vi "ILCTest.vi"() -> ()   [LabVIEW 2016]
uses:
  Common_RT_HPILC/DataTypes/HPTelemetry.ctl
  Stats.ctl
  Common_RT_Modbus/DataTypes/RxFrame.ctl
  Common_RT_HealthAndStatus/RTHealthAndStatus/RTHealthAndStatus.lvclass
  MyHealthAndStatusReadFIFO/MyHealthAndStatusReadFIFO.lvclass
  D:/Code/Common_RT_FPGA/IReadU32FIFO/IReadU32FIFO.lvclass
  MyHealthAndStatusWriteFIFO/MyHealthAndStatusWriteFIFO.lvclass
  D:/Code/Common_RT_FPGA/IWriteU64FIFO/IWriteU64FIFO.lvclass
  ModbusFactory/ModbusFactory.lvclass
  D:/Code/Common_RT_Modbus/IModbusFactory/IModbusFactory.lvclass
  SubnetFactory/SubnetFactory.lvclass
  Subnet/DataTypes/SubnetSettings.ctl
  Common_RT_HPILC/DataTypes/HPSettings.ctl
  Common_RT_ILC/DataTypes/ILCSettings.ctl
  Common_RT_Modbus/IModbusFactory/IModbusFactory.lvclass
  Common_RT_MTILC/DataTypes/MTSettings.ctl
  Common_RT_MDILC/DataTypes/MDSettings.ctl
  Common_RT_MIILC/DataTypes/MISettings.ctl
  Accel1TimestampFIFO/Accel1TimestampFIFO.lvclass
  D:/Code/Common_RT_FPGA/IReadU64FIFO/IReadU64FIFO.lvclass
  Scratch/RTMonitorAccelerometer/MonitorAccelerometer/MonitorAccelerometer.lvclass
  Accel1Channel0FIFO/Accel1Channel0FIFO.lvclass
  D:/Code/Common_RT_FPGA/IReadSGLFIFO/IReadSGLFIFO.lvclass
  Accel1Channel1FIFO/Accel1Channel1FIFO.lvclass
  Accel1Channel2FIFO/Accel1Channel2FIFO.lvclass
  Accel1Channel2FIFO/Accel1Channel2FIFO.lvclass/Accel1Channel2FIFO.ctl
  Accel1Channel1FIFO/Accel1Channel1FIFO.lvclass/Accel1Channel1FIFO.ctl
  Accel1Channel0FIFO/Accel1Channel0FIFO.lvclass/Accel1Channel0FIFO.ctl
  Accel1TimestampFIFO/Accel1TimestampFIFO.lvclass/Accel1TimestampFIFO.ctl
  Scratch/RTMonitorAccelerometer/MonitorAccelerometer/MonitorAccelerometer.lvclass/MonitorAccelerometer.ctl
  ModbusFactory/ModbusFactory.lvclass/ModbusFactory.ctl
  MyHealthAndStatusWriteFIFO/MyHealthAndStatusWriteFIFO.lvclass/MyHealthAndStatusWriteFIFO.ctl
  MyHealthAndStatusReadFIFO/MyHealthAndStatusReadFIFO.lvclass/MyHealthAndStatusReadFIFO.ctl
  Common_RT_HealthAndStatus/RTHealthAndStatus/RTHealthAndStatus.lvclass/RTHealthAndStatus.ctl
  Subnet/Subnet.lvclass/Subnet.ctl
  Common_RT_HPILC/HPILC/HPILC.lvclass/HPILC.ctl
  <vilib>/Platform/TimedLoop/XDataNode/timing_clust.ctl
  <vilib>/Platform/TimedLoop/XDataNode/nitl_modes.ctl
  <vilib>/Platform/TimedLoop/XDataNode/wakeup.ctl
  Common_RT_MIILC/MIILC/MIILC.lvclass/MIILC.ctl
  Common_RT_MDILC/MDILC/MDILC.lvclass/MDILC.ctl
  Common_RT_MTILC/MTILC/MTILC.lvclass/MTILC.ctl
  <vilib>/FPGAPlugInAG/cRIO-9038/niLvFpga_Open_cRIO-9038.vi
  <vilib>/rvi/interface/common/dynamic/niFpgaDynamicAddResources.vi
  <vilib>/FPGAPlugInAG/Dynamic/niLvFpga_Abort_Dynamic.vi
  <vilib>/FPGAPlugInAG/Dynamic/niLvFpga_Reset_Dynamic.vi
  <vilib>/FPGAPlugInAG/Dynamic/niLvFpga_Run_Dynamic.vi
  <vilib>/Utility/error.llb/Error Cluster From Error Code.vi
  <vilib>/rvi/errors/niLvFpgaAdjustHostInterfaceError.vi
  <vilib>/Instr/_visa.llb/VISA Configure Serial Port (Instr).vi
  <vilib>/FPGAPlugInAG/Dynamic/niLvFpga_Close_Dynamic.vi
  <vilib>/rvi/interface/nirviOpenFPGA/nirviOpenFPGA.xnode
  FPGA Bitfiles/modbus1Port.lvbitx
  FPGA/main.vi
  <vilib>/rvi/interface/nirviMethod/nirviMethod.xnode
  <vilib>/platform/TimedLoop/XDataNode/XDataNode.xnode
  <vilib>/rvi/interface/nirviCloseFPGA/nirviCloseFPGA.xnode
  Subnet/Subnet.lvclass
  Common_RT_ILC/RTILC.lvlib
  Common_RT_HPILC/RTHPILC.lvlib
  Common_RT_HPILC/HPILC/HPILC.lvclass
  <vilib>/rvi/errors/niLvFpgaMergeErrorWithErrorCode.vi
  <vilib>/FPGAPlugInAG/Dynamic/niLvFpga_ReadFifo_Dynamic.vi
  Common_RT_MTILC/MTILC/MTILC.lvclass
  Common_RT_MDILC/MDILC/MDILC.lvclass
  Common_RT_MIILC/MIILC/MIILC.lvclass
  Common_RT_MIILC/RTMIILC.lvlib
  Common_RT_MDILC/RTMDILC.lvlib
  Common_RT_MTILC/RTMTILC.lvlib
  <vilib>/Platform/TimedLoop/XDataNode/XDNodeRunTimeDep.lvlib
  Common_RT_Modbus/RTModbus.lvlib
panel:
  out "unsigned byte array":u8[](array[numeric])
  out "XY Graph":cluster{"Timestamp":dbl[], "Channel2":sgl[]}[](graph)
  out "Timestamp":u64[](array[numeric])
  out "CRC":T1[](array[typedef]) {"Data" format="%02x"}
  out "Displacement":T2(graph)
  out "Inclination":cluster{"Angle":sgl}(graph)
  out "Temperature":T3(graph)
  out "output cluster":T4={"MinLoopTime"=99999.0, "MaxLoopTime"=-99999.0}
  in  "Steps":i32=1
  out "Loop Time":cluster{u32, "Messages":i32}(graph)
  out "InvalidCRCs":i32
  out "Actuator Telemetry":T5[](array[typedef])
  out "Encoder":T6(graph)
  in  "Stop":bool
  out "Port 1 Status Bits":u64 format="%016b"
  out "error out":errorcluster
  out "Port 1 Frames Received":i64
  out "Port 1 Bytes Received":i64
  out "Port 1 Frames Transmitted":i64
  out "Port 1 Bytes Transmitted":i64
  # "Port 1 = Modbus"
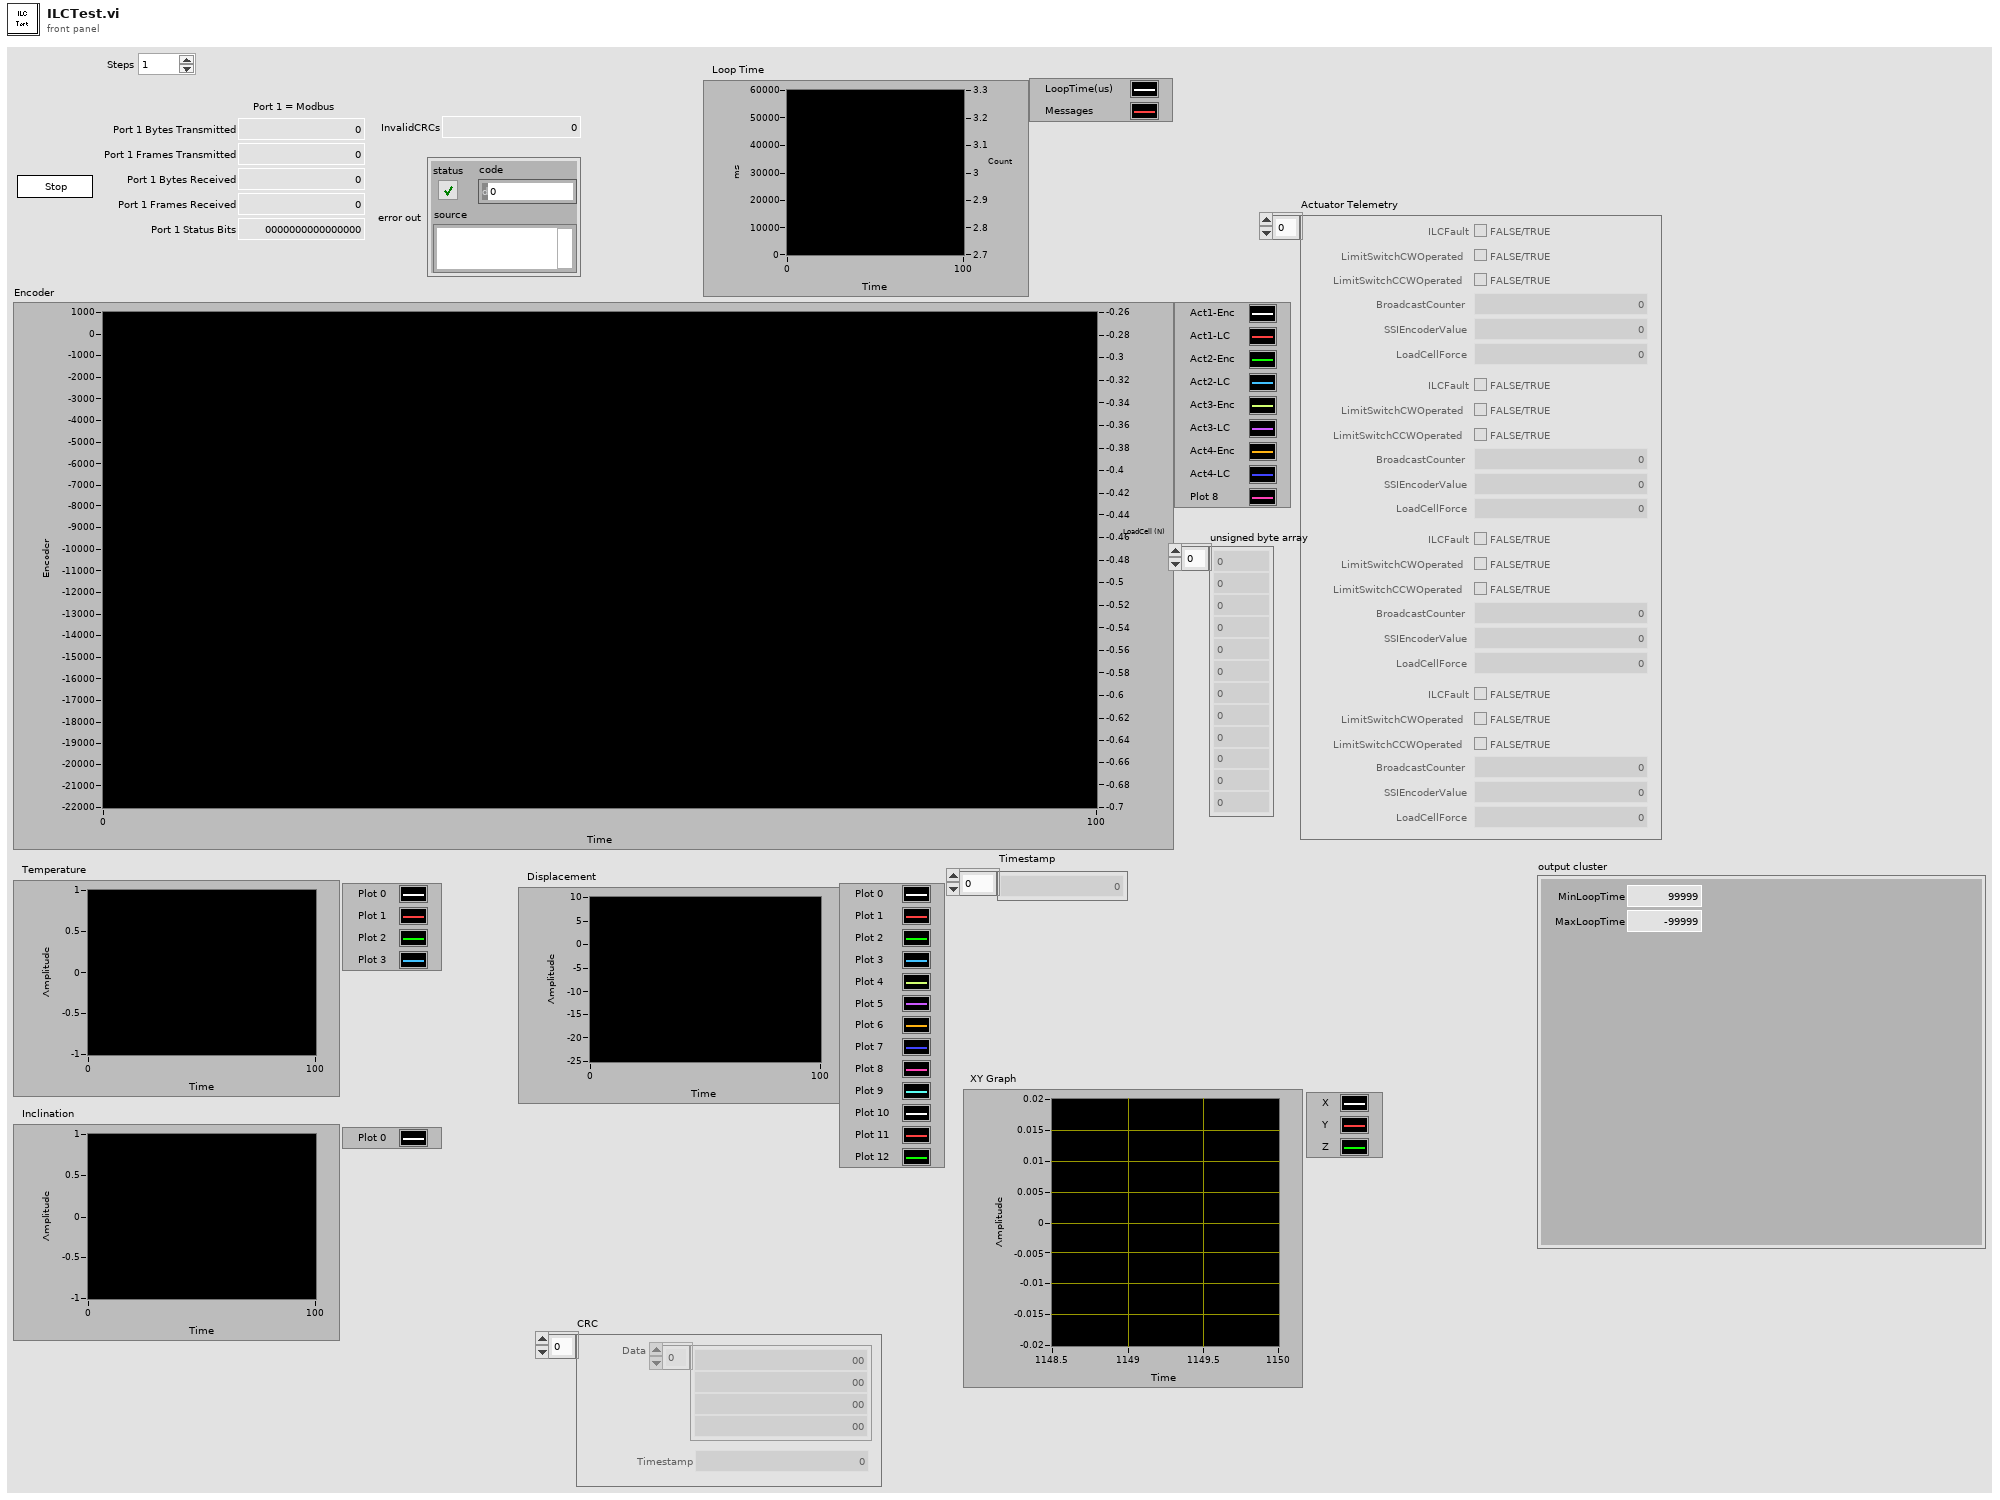
[diagram p1: front panel]
types:
  T1 = typedef "RTModbus.lvlib/RxFrame.ctl" = cluster{"Data":u8[], "Timestamp":u64}
  T2 = cluster{"Displacement1":sgl, "Displacement1":sgl, "Displacement1":sgl, "Displacement1":sgl, "Displacement1":sgl, "Displacement1":sgl}
  T3 = cluster{"Temperature1":sgl, "Temperature1":sgl, "Temperature1":sgl, "Temperature1":sgl}
  T4 = typedef "Stats.ctl" = cluster{"MinLoopTime":dbl, "MaxLoopTime":dbl}
  T5 = typedef "RTHPILC.lvlib/HPTelemetry.ctl" = cluster{"ILCFault":bool, "LimitSwitchCWOperated":bool, "LimitSwitchCCWOperated":bool, "BroadcastCounter":u8, "SSIEncoderValue":i32, "LoadCellForce":sgl}
  T6 = cluster{"[0]":dbl, "[1]":dbl, "[2]":dbl, "[3]":dbl, "[4]":dbl, "[5]":dbl, "[6]":dbl, "[7]":dbl, "[8]":dbl}
  T7 = typedef "RTMIILC.lvlib/MISettings.ctl" = cluster{"ILCSettings":T8, "ID":i16}
  T8 = typedef "RTILC.lvlib/ILCSettings.ctl" = cluster{"Subnet":u8, "Address":u8}
  T9 = typedef "RTMDILC.lvlib/MDSettings.ctl" = cluster{"ILCSettings":T8, "ID":i16}
  T10 = typedef "RTMTILC.lvlib/MTSettings.ctl" = cluster{"ILCSettings":T8, "ID":i16}
  T11 = typedef "RTHPILC.lvlib/HPSettings.ctl" = cluster{"ILCSettings":T8, "ID":i16, "ReferencePosition":i32}
  T12 = enum16{"open", "replace", "create", "open or create", "replace or create", "replace or create with confirmation"}
  T13 = typedef "XDNodeRunTimeDep.lvlib/timing_clust.ctl" = cluster{"Expected End [f-1]":u64, "Actual End [f-1]":u64, "Finished Late? [f-1]":bool, "Expected End [i-1]":u64, "Actual End [i-1]":u64, "Finished Late? [i-1]":bool, "Expected Start [i]":u64, "Actual Start [i]":u64, "Expected Start [f]":u64, "Actual Start [f]":u64, "Source Name":string, "Structure Name":string, "Period":i64, "Deadline":i64, "Offset":i64, "Start":i64, "Priority":i32, "Timeout":i32, "Mode":T14, "Wakeup Reason":T15, "Error":errorcluster, "Source Type":string, "Secondary Source Type":string, "Global End Time":u64, "Global Start Time":u64, "Frame Duration":u64, "Iteration Duration":u64, "Assigned CPU":i32, "I/O Scan Engine Mode":u32}
  T14 = typedef "XDNodeRunTimeDep.lvlib/nitl_modes.ctl" = enum32{"No Change", "Process missed periods, maintain original phase", "Discard missed periods, maintain original phase", "Process missed periods, ignore original phase", "Discard missed periods, ignore original phase"}
  T15 = typedef "XDNodeRunTimeDep.lvlib/wakeup.ctl" = enum32{"Normal", "Aborted", "Asynchronous wakeup", "Timing source error", "Timed loop error", "Timeout"}
  T16 = typedef "SubnetSettings.ctl" = cluster{"HPs":T11[], "ModbusFactory":refnum<class "IModbusFactory.lvclass">, "Port":i32, "MTs":T10[], "MDs":T9[], "MIs":T7[]}
  T17 = typedef "SubnetData.ctl" = cluster{"SubnetConstants":T18, "SubnetCommand":T21, "SubnetTelemetry":T22}
  T18 = typedef "SubnetConstants.ctl" = cluster{"Modbus":refnum<class "IModbus.lvclass">, "HPs":refnum<class "HPILC.lvclass">[], "AddressToActuator":T19[], "MTs":refnum<class "MTILC.lvclass">[], "MDs":refnum<class "MDILC.lvclass">[], "MIs":refnum<class "MIILC.lvclass">[]}
  T19 = typedef "ILCIndexData.ctl" = cluster{"ILCTypes":T20, "Index":i32}
  T20 = typedef "ILCTypes.ctl" = enum16{"Undefined", "SAA", "DAA", "HP", "MT", "MD", "MI"}
  T21 = typedef "SubnetCommand.ctl" = cluster{"BroadcastCounter":u8}
  T22 = typedef "SubnetTelemetry.ctl" = cluster{"BytesTransmitted":u32, "FramesTransmitted":u32, "BytesReceived":u32, "FramesReceived":u32, "TxInternalFIFOOverflow":bool, "InvalidInstruction":bool, "WaitForRxFrameTimeout":bool, "StartBitError":bool, "StopBitError":bool, "RxDataFIFOOverflow":bool}
  T23 = typedef "RTHPILC.lvlib/HPData.ctl" = cluster{"Constants":T24, "Command":T25, "Telemetry":T5, "Responses":T26, "Timings":T28}
  T24 = typedef "RTHPILC.lvlib/HPConstants.ctl" = cluster{"ID":i16, "ReferencePosition":i32}
  T25 = typedef "RTHPILC.lvlib/HPCommand.ctl" = cluster{"Steps":i8}
  T26 = typedef "RTHPILC.lvlib/HPResponses.ctl" = cluster{"StepMotor":T27, "ForceAndStatus":T27}
  T27 = typedef "RTModbus.lvlib/ExceptionCodes.ctl" = u16
  T28 = typedef "RTHPILC.lvlib/HPTimings.ctl" = cluster{"BroadcastStepMotor":u32, "ForceAndStatus":u32, "FreezeSensorValues":u32, "StepMotor":u32}
  T29 = typedef "RTMTILC.lvlib/MTData.ctl" = cluster{"Constants":T30, "Telemetry":T31, "Responses":T32, "Timings":T33}
  T30 = typedef "RTMTILC.lvlib/MTConstants.ctl" = cluster{"ID":i16}
  T31 = typedef "RTMTILC.lvlib/MTTelemetry.ctl" = cluster{"Temperature":sgl[]}
  T32 = typedef "RTMTILC.lvlib/MTResponses.ctl" = cluster{"Temperature":T27}
  T33 = typedef "RTMTILC.lvlib/MTTimings.ctl" = cluster{"Temperature":u32}
  T34 = typedef "RTMDILC.lvlib/MDData.ctl" = cluster{"Constants":T35, "Telemetry":T36, "Responses":T37, "Timings":T38}
  T35 = typedef "RTMDILC.lvlib/MDConstants.ctl" = cluster{"ID":i16}
  T36 = typedef "RTMDILC.lvlib/MDTelemetry.ctl" = cluster{"Displacement":sgl[]}
  T37 = typedef "RTMDILC.lvlib/MDResponses.ctl" = cluster{"Displacement":T27}
  T38 = typedef "RTMDILC.lvlib/MDTimings.ctl" = cluster{"Displacement":u32}
  T39 = typedef "RTMIILC.lvlib/MIData.ctl" = cluster{"Constants":T40, "Telemetry":T41, "Responses":T42, "Timings":T43}
  T40 = typedef "RTMIILC.lvlib/MIConstants.ctl" = cluster{"ID":i16}
  T41 = typedef "RTMIILC.lvlib/MITelemetry.ctl" = cluster{"Angle":sgl}
  T42 = typedef "RTMIILC.lvlib/MIResponses.ctl" = cluster{"Inclination":T27}
  T43 = typedef "RTMIILC.lvlib/MITimings.ctl" = cluster{"Inclination":u32}
  T44 = typedef "RTMonitorAccelerometer.lvlib/MonitorAccelerometerData.ctl" = cluster{"Timestamp":dbl[], "Channel0":sgl[], "Channel1":sgl[], "Channel2":sgl[]}
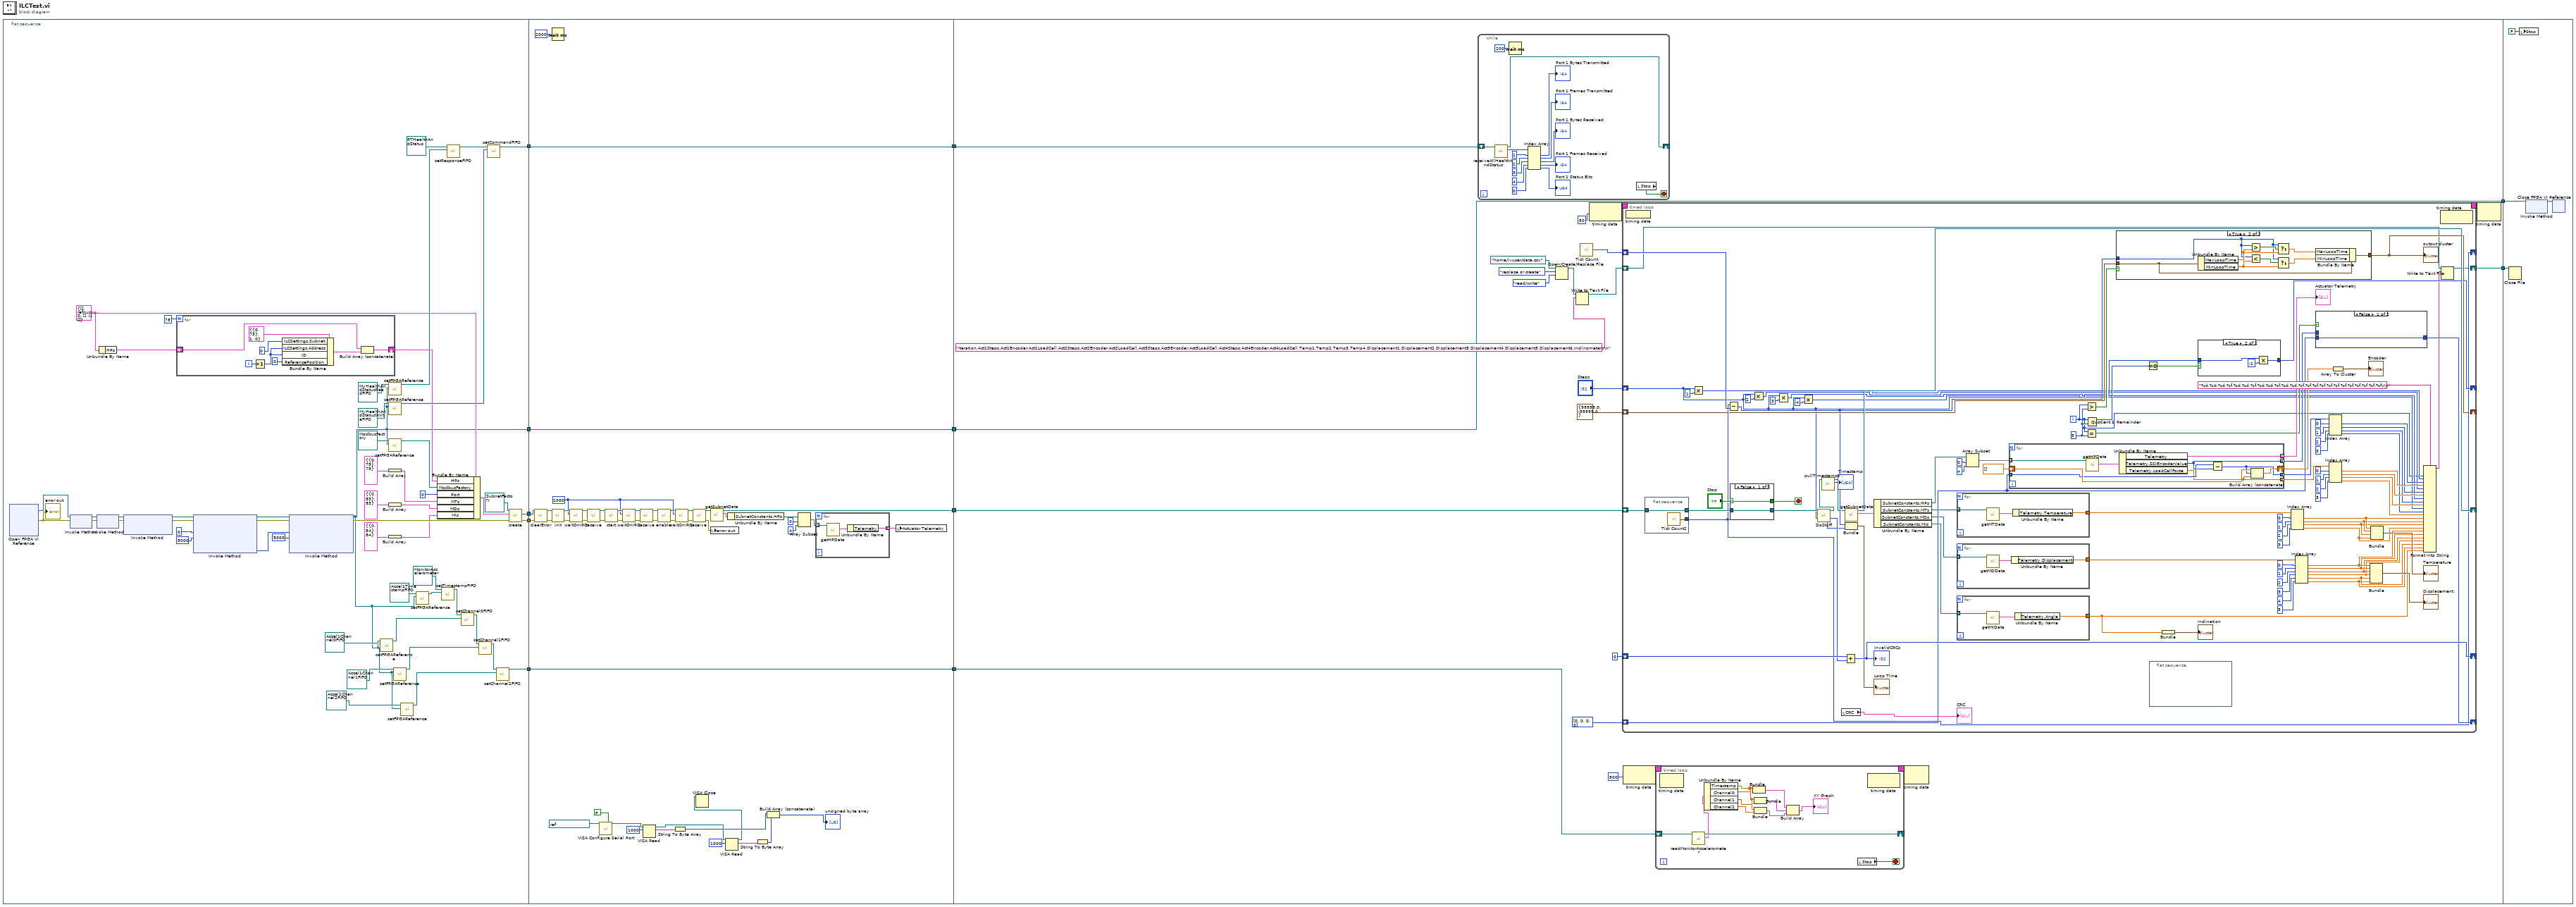
[diagram p0: block diagram]
diagram:
  n1 = flat-sequence {
    tunnel: [w13] -> w11
    tunnel: [w61] -> w8
    tunnel: [w48] -> w6
    tunnel: [w33] -> w4
    tunnel: [w12] -> w2
    tunnel: w11 -> [w118]
    tunnel: [w118] -> w10
    tunnel: w8 -> [w116]
    tunnel: [w116] -> w7
    tunnel: w6 -> [w94]
    tunnel: [w96] -> w5
    tunnel: w4 -> [w86]
    tunnel: w2 -> [w85]
    tunnel: [w85] -> w1
    tunnel: w10 -> [w142]
    tunnel: [w142] -> w9
    tunnel: w7 -> [w143]
    tunnel: w5 -> [w141]
    tunnel: [w132] -> w3
    tunnel: w1 -> [w122]
    tunnel: w9 -> [w324]
    tunnel: w3 -> [w322]
    frame #0 {
      w53 = T16 {"HPs"=[], "ModbusFactory"=refnum, "Port"=0, "MTs"=[], "MDs"=[], "MIs"=[]} ("SubnetSettings")
      n2 = xnode "Open FPGA VI Reference"() -> ("FPGA VI Reference Out"=w55:refnum<k20>, "error out"=w35:errorcluster)  [unwired: 2 in]
      "error out" <- w35
      n3 = xnode "Invoke Method"("FPGA VI Reference In"=w55, "error in"=w35) -> ("FPGA VI Reference Out"=w64:refnum<k20>, "error out"=w56:errorcluster)
      n4 = xnode "Invoke Method"("FPGA VI Reference In"=w64, "error in"=w56) -> ("FPGA VI Reference Out"=w41:refnum<k20>, "error out"=w39:errorcluster)
      n5 = Unbundle By Name(w53) -> ("HPs"=w37:T11[])
      n6 = xnode "Invoke Method"("FPGA VI Reference In"=w41, "error in"=w39) -> ("FPGA VI Reference Out"=w40:refnum<k20>, "error out"=w38:errorcluster)  [unwired: 1 in]
      n7 = for {
        N: 78 -> [_]
        shift-right: [w66] -> w36
        shift-left: w37 -> [w67]
        i -> [w71]
        n8 = Increment(x=w71) -> (x+1=w65:i32)
        n9 = Bundle By Name(cluster=T11 {"ILCSettings"={"Subnet"=0, "Address"=73}, "ID"=1, "ReferencePosition"=0} ("HPSettings"), "ILCSettings.Subnet"=u8 0, "ILCSettings.Address"=w65, "ID"=w65, "ReferencePosition"=0) -> (w68:T11)
        n10 = Build Array (concatenate)(w67, w68) -> (w66:T11[])
      }
      n11 = xnode "Invoke Method"("FPGA VI Reference In"=w40, "error in"=w38, "Number of Elements"=u32 0, "Timeout (ms)"=5000) -> ("FPGA VI Reference Out"=w44:refnum<k20>, "error out"=w42:errorcluster, "Elements Remaining"=w45:u32)  [unwired: 1 out]
      n12 = xnode "Invoke Method"("FPGA VI Reference In"=w44, "error in"=w42, "Number of Elements"=w45, "Timeout (ms)"=5000) -> ("FPGA VI Reference Out"=w13:refnum<k20>, "error out"=w34:errorcluster)  [unwired: 2 out]
      n13 = call "setFPGAReference.vi"("FPGAReference"=w13, "MyHealthAndStatusReadFIFO in"=refnum<class "Accel1Channel0FIFO.lvclass"> refnum ("Accel1Channel0FIFO.lvclass")) -> ("MyHealthAndStatusReadFIFO out"=w18:refnum<class "Accel1Channel0FIFO.lvclass">)  [unwired: 9 in]
      n14 = call "setFPGAReference.vi"("FPGAReference"=w13, "MyHealthAndStatusReadFIFO in"=refnum<class "MyHealthAndStatusReadFIFO.lvclass"> refnum ("MyHealthAndStatusReadFIFO.lvclass")) -> ("MyHealthAndStatusReadFIFO out"=w59:refnum<class "MyHealthAndStatusReadFIFO.lvclass">)  [unwired: 9 in]
      n15 = call "setFPGAReference.vi"("FPGAReference"=w13, "MyHealthAndStatusWriteFIFO in"=refnum<class "MyHealthAndStatusWriteFIFO.lvclass"> refnum ("MyHealthAndStatusWriteFIFO.lvclass")) -> ("MyHealthAndStatusWriteFIFO out"=w57:refnum<class "MyHealthAndStatusWriteFIFO.lvclass">)  [unwired: 9 in]
      n16 = call "setFPGAReference.vi"("FPGAReference"=w13, "ModbusFactory in"=refnum<class "ModbusFactory.lvclass"> refnum ("ModbusFactory.lvclass")) -> ("ModbusFactory out"=w51:refnum<class "ModbusFactory.lvclass">)  [unwired: 9 in]
      n17 = Build Array(T10 {"ILCSettings"={"Subnet"=0, "Address"=79}, "ID"=79} ("MTSettings")) -> (w26:T10[])
      n18 = Build Array(T9 {"ILCSettings"={"Subnet"=0, "Address"=83}, "ID"=83} ("MDSettings")) -> (w27:T9[])
      n19 = Build Array(T7 {"ILCSettings"={"Subnet"=0, "Address"=84}, "ID"=84} ("MISettings")) -> (w28:T7[])
      n20 = call "setFPGAReference.vi"("FPGAReference"=w13, "MyHealthAndStatusReadFIFO in"=refnum<class "Accel1Channel1FIFO.lvclass"> refnum ("Accel1Channel1FIFO.lvclass")) -> ("MyHealthAndStatusReadFIFO out"=w16:refnum<class "Accel1Channel1FIFO.lvclass">)  [unwired: 9 in]
      n21 = call "setFPGAReference.vi"("FPGAReference"=w13, "MyHealthAndStatusReadFIFO in"=refnum<class "Accel1Channel2FIFO.lvclass"> refnum ("Accel1Channel2FIFO.lvclass")) -> ("MyHealthAndStatusReadFIFO out"=w14:refnum<class "Accel1Channel2FIFO.lvclass">)  [unwired: 9 in]
      n22 = call "setFPGAReference.vi"("FPGAReference"=w13, "MyHealthAndStatusReadFIFO in"=refnum<class "Accel1TimestampFIFO.lvclass"> refnum ("Accel1TimestampFIFO.lvclass")) -> ("MyHealthAndStatusReadFIFO out"=w22:refnum<class "Accel1TimestampFIFO.lvclass">)  [unwired: 9 in]
      n23 = Bundle By Name(cluster=w53, "HPs"=w36, "ModbusFactory"=w51, "Port"=0, "MTs"=w26, "MDs"=w27, "MIs"=w28) -> (w50:T16)
      n24 = call "setTimestampFIFO.vi"("TimestampFIFO"=w22, "MonitorAccelerometer in"=refnum<class "MonitorAccelerometer.lvclass"> refnum ("RTMonitorAccelerometer.lvlib:MonitorAccelerometer.lvclass")) -> ("MonitorAccelerometer out"=w23:refnum<class "MonitorAccelerometer.lvclass">)  [unwired: 9 in]
      n25 = call "setResponseFIFO.vi"("ReadU32FIFO"=w59, "RTHealthAndStatus in"=refnum<class "RTHealthAndStatus.lvclass"> refnum ("RTHealthAndStatus.lvlib:RTHealthAndStatus.lvclass")) -> ("RTHealthAndStatus out"=w62:refnum<class "RTHealthAndStatus.lvclass">)  [unwired: 9 in]
      n26 = call "setChannel0FIFO.vi"("Channel0FIFO"=w18, "MonitorAccelerometer in"=w23) -> ("MonitorAccelerometer out"=w21:refnum<class "MonitorAccelerometer.lvclass">)  [unwired: 9 in]
      n27 = call "setChannel1FIFO.vi"("Channel1FIFO"=w16, "MonitorAccelerometer in"=w21) -> ("MonitorAccelerometer out"=w20:refnum<class "MonitorAccelerometer.lvclass">)  [unwired: 9 in]
      n28 = call "setCommandFIFO.vi"("WriteU64FIFO"=w57, "RTHealthAndStatus in"=w62) -> ("RTHealthAndStatus out"=w61:refnum<class "RTHealthAndStatus.lvclass">)  [unwired: 9 in]
      n29 = call "setChannel2FIFO.vi"("Channel2FIFO"=w14, "MonitorAccelerometer in"=w20) -> ("MonitorAccelerometer out"=w12:refnum<class "MonitorAccelerometer.lvclass">)  [unwired: 9 in]
      n30 = call "create.vi"("error in (no error)"=w34, "SubnetSettings"=w50, "SubnetFactory in"=refnum<class "SubnetFactory.lvclass"> refnum ("SubnetFactory.lvclass")) -> ("error out"=w33:errorcluster, "Subnet"=w48:refnum<class "Subnet.lvclass">)  [unwired: 6 in, 1 out]
    }
    frame #1 {
      w99 = 1000 ("Timeout (ms)")
      n31 = call-dynamic "clearError.vi"("error in (no error)"=w86, "Subnet in"=w94) -> ("error out"=w92:errorcluster, "Subnet out"=w93:refnum<class "Subnet.lvclass">)  [unwired: 8 in]
      n32 = Wait (ms)(milliseconds to wait=u32 2000) -> ()  [unwired: 1 out]
      n33 = call-dynamic "init.vi"("error in (no error)"=w92, "Subnet in"=w93) -> ("error out"=w112:errorcluster, "Subnet out"=w115:refnum<class "Subnet.lvclass">)  [unwired: 8 in]
      n34 = call-dynamic "waitOnIRQ.vi"("error in (no error)"=w112, "Timeout (ms)"=w99, "Subnet in"=w115) -> ("error out"=w113:errorcluster, "Subnet out"=w114:refnum<class "Subnet.lvclass">)  [unwired: 7 in]
      n35 = call-dynamic "receive.vi"("Subnet in"=w114, "error in (no error)"=w113) -> ("Subnet out"=w111:refnum<class "Subnet.lvclass">, "error out"=w109:errorcluster)  [unwired: 8 in, 4 out]
      n36 = call-poly "VISA Configure Serial Port"("VISA resource name"=refnum<visa-resource-name> "ASRL1::INSTR", "Enable Termination\nChar (T)"=FALSE ("Enable Termination\nChar (T)")) -> ("VISA resource name out"=w82:refnum<visa-resource-name>)  [unwired: 12 in, 1 out]
      n37 = call-dynamic "start.vi"("error in (no error)"=w109, "Subnet in"=w111) -> ("error out"=w108:errorcluster, "Subnet out"=w110:refnum<class "Subnet.lvclass">)  [unwired: 8 in]
      n38 = call-dynamic "waitOnIRQ.vi"("error in (no error)"=w108, "Timeout (ms)"=w99, "Subnet in"=w110) -> ("error out"=w106:errorcluster, "Subnet out"=w107:refnum<class "Subnet.lvclass">)  [unwired: 7 in]
      n39 = call-dynamic "receive.vi"("Subnet in"=w107, "error in (no error)"=w106) -> ("Subnet out"=w105:refnum<class "Subnet.lvclass">, "error out"=w104:errorcluster)  [unwired: 8 in, 4 out]
      n40 = VISA Read(VISA resource name=w82, byte count=u32 1000) -> (VISA resource name out=w77:refnum<visa-resource-name>, read buffer=w80:string)  [unwired: 1 in, 2 out]
      n41 = call-dynamic "enable.vi"("error in (no error)"=w104, "Subnet in"=w105) -> ("error out"=w100:errorcluster, "Subnet out"=w103:refnum<class "Subnet.lvclass">)  [unwired: 8 in]
      n42 = String To Byte Array(string=w80) -> (unsigned byte array=w76:u8[])
      n43 = call-dynamic "waitOnIRQ.vi"("error in (no error)"=w100, "Timeout (ms)"=w99, "Subnet in"=w103) -> ("error out"=w102:errorcluster, "Subnet out"=w101:refnum<class "Subnet.lvclass">)  [unwired: 7 in]
      n44 = call-dynamic "receive.vi"("Subnet in"=w101, "error in (no error)"=w102) -> ("Subnet out"=w98:refnum<class "Subnet.lvclass">, "error out"=w95:errorcluster)  [unwired: 8 in, 4 out]
      n45 = call "getSubnetData.vi"("Subnet in"=w98) -> ("SubnetData"=w97:T17, "Subnet out"=w96:refnum<class "Subnet.lvclass">)  [unwired: 9 in]
      n46 = local write "error out"(w95) -> ()
      n47 = VISA Read(VISA resource name=w77, byte count=u32 1000) -> (VISA resource name out=w73:refnum<visa-resource-name>, read buffer=w79:string)  [unwired: 1 in, 2 out]
      n48 = VISA Close(VISA resource name=w73) -> ()  [unwired: 1 in, 1 out]
      n49 = Unbundle By Name(w97) -> ("SubnetConstants.HPs"=w91:refnum<class "HPILC.lvclass">[])
      n50 = String To Byte Array(string=w79) -> (unsigned byte array=w75:u8[])
      n51 = Build Array (concatenate)(w76, w75) -> (→"unsigned byte array":u8[])
      n52 = Array Subset(array=w91, index=0, length=4) -> (w88:refnum<class "HPILC.lvclass">[])
      n53 = for {
        tunnel: w88 -> [w121] mode=indexing
        tunnel: [w119] -> w87 mode=indexing
        n54 = call "getHPData.vi"("HPILC in"=w121) -> ("HPData"=w120:T23)  [unwired: 9 in, 1 out]
        n55 = Unbundle By Name(w120) -> ("Telemetry"=w119:T5)
      }
      n56 = local write "Actuator Telemetry"(w87) -> ()
    }
    frame #2 {
      n57 = while {
        shift-right: [w319] -> _
        shift-left: w143 -> [w320]
        stop <- w307 stop-if-true
        n58 = call "receiveAllHealthAndStatus.vi"("RTHealthAndStatus in"=w320) -> ("Data"=w314:u32[], "RTHealthAndStatus out"=w319:refnum<class "RTHealthAndStatus.lvclass">)  [unwired: 8 in, 1 out]
        n59 = Wait (ms)(milliseconds to wait=u32 200) -> ()  [unwired: 1 out]
        n60 = Index Array(array=w314, index #1=1 ("index"), index #2=2 ("index"), index #3=3 ("index"), index #4=4 ("index"), index #5=0 ("index")) -> (element #1=→"Port 1 Bytes Transmitted":u32, element #2=→"Port 1 Frames Transmitted":u32, element #3=→"Port 1 Bytes Received":u32, element #4=→"Port 1 Frames Received":u32, element #5=→"Port 1 Status Bits":u32)
        n61 = local read "Stop"() -> (w307:bool)
      }
      n62 = Open/Create/Replace File(file path (use dialog)=path "/home/lvuser/data.csv", operation (0:open)=T12."replace or create", access (0:read/write)=enum16{"read/write", "read-only", "write-only"}."read/write") -> (refnum out=w131:refnum<file>)  [unwired: 3 in, 2 out]
      n63 = Write to Text File(file (use dialog)=w131, text="Iteration,Act1Steps,Act1Encoder,Act1LoadCell,Act2Steps,Act2Encoder,Act2LoadCell,Act3Steps,Act3Encoder,Act3LoadCell,Act4Steps,Act4Encoder,Act4LoadCell,Temp1,Temp2,Temp3,Temp4,Displacement1,Displacement2,Displacement3,Displacement4,Displacement5,Displacement6,Inclinometer\r\n" ("format string")) -> (refnum out=w130:refnum<file>)  [unwired: 2 in, 2 out]
      n64 = call "Tick Count"() -> ("Tick Count(uSec)"=w139:u32)
      n65 = node-c288(i64 50 ("Period")) -> (w128:T13)
      n66 = timed-loop {
        shift-right: [w256] -> _
        shift-left: w141 -> [w237]
        shift-right: [w245] -> _
        shift-left: "Steps" -> [w207]
        shift-right: [w249] -> _
        shift-left: 0 -> [w250]
        shift-right: [w235] -> _
        shift-left: w139 -> [w248]
        shift-right: [w242] -> _
        shift-left: i32[] [0, 0, 0, 0] -> [w241]
        shift-right: [w228] -> _
        shift-left: T4 {"MinLoopTime"=99999.0, "MaxLoopTime"=-99999.0} ("Stats") -> [w229]
        shift-right: [w167] -> w132
        shift-left: w130 -> [w168]
        timing: w128 -> [_]
        timing-out: [_] -> w127
        i -> [w162]
        stop <- w259 stop-if-true
        w230 = 5 ("y")
        n67 = node-c288() -> ()  [unwired: 1 in]
        n68 = flat-sequence {
          tunnel: w237 -> [w283]
          tunnel: [w283] -> w236
          tunnel: [w282] -> w235
          frame #0 {
            n69 = call "Tick Count2"() -> ("Tick Count(uSec)"=w282:u32)
          }
        }
        n70 = Multiply(x=w207, y=1) -> (x*y=w197:i32)
        n71 = Subtract(x=w235, y=w248) -> (x-y=w227:u32)
        n72 = case shown="False" "Stop" {
          selector: "Stop" -> [w299 w301]
          tunnel: [w299 w301] -> w259
          tunnel: w236 -> [w300 w302]
          tunnel: [w300 w302] -> w258
          frame False {
          }
          frame True {
          }
        }
        n73 = Multiply(x=w207, y=2) -> (x*y=w189:i32)
        n74 = Multiply(x=w207, y=3) -> (x*y=w186:i32)
        n75 = Multiply(x=w207, y=4) -> (x*y=w183:i32)
        n76 = call "DoStuff.vi"("Subnet in"=w258, "Steps"=w207) -> ("Subnet out"=w166:refnum<class "Subnet.lvclass">, "InvalidCRC"=w239:i32, "Messages"=w238:i32)  [unwired: 7 in, 4 out]
        n77 = call-dynamic "pullTimestamps.vi"("Subnet in"=w166) -> ("Timestamp"=→"Timestamp":u64[], "Subnet out"=w165:refnum<class "Subnet.lvclass">)  [unwired: 8 in, 1 out]
        n78 = local read "CRC"() -> (→"CRC":T1[])
        n79 = Add(x=w250, y=w239) -> (x+y=w249:i32)
        "InvalidCRCs" <- w249
        n80 = Bundle(w227, "Messages"=w238) -> (→"Loop Time":cluster{u32, "Messages":i32})  [unwired: 1 in]
        n81 = call "getSubnetData.vi"("Subnet in"=w165) -> ("SubnetData"=w257:T17, "Subnet out"=w256:refnum<class "Subnet.lvclass">)  [unwired: 9 in]
        n82 = Unbundle By Name(w257) -> ("SubnetConstants.HPs"=w253:refnum<class "HPILC.lvclass">[], "SubnetConstants.MTs"=w226:refnum<class "MTILC.lvclass">[], "SubnetConstants.MDs"=w225:refnum<class "MDILC.lvclass">[], "SubnetConstants.MIs"=w224:refnum<class "MIILC.lvclass">[])
        n83 = for {
          tunnel: w226 -> [w271] mode=indexing
          tunnel: [w269] -> w223
          n84 = call "getMTData.vi"("MTILC in"=w271) -> ("MTData"=w270:T29)  [unwired: 9 in, 1 out]
          n85 = Unbundle By Name(w270) -> ("Telemetry.Temperature"=w269:sgl[])
        }
        n86 = for {
          tunnel: w225 -> [w267] mode=indexing
          tunnel: [w266] -> w216
          n87 = call "getMDData.vi"("MDILC in"=w267) -> ("MDData"=w268:T34)  [unwired: 9 in, 1 out]
          n88 = Unbundle By Name(w268) -> ("Telemetry.Displacement"=w266:sgl[])
        }
        n89 = for {
          tunnel: w224 -> [w265] mode=indexing
          tunnel: [w263] -> w170
          n90 = call "getMIData.vi"("MIILC in"=w265) -> ("MIData"=w264:T39)  [unwired: 9 in, 1 out]
          n91 = Unbundle By Name(w264) -> ("Telemetry.Angle"=w263:sgl)
        }
        n92 = Array Subset(array=w253, index=0, length=4) -> (w252:refnum<class "HPILC.lvclass">[])
        n93 = for {
          tunnel: w252 -> [w298] mode=indexing
          shift-right: [w295] -> w234
          shift-left: dbl[] [] -> [w296]
          tunnel: [w294] -> w244 mode=indexing
          tunnel: [w292] -> w243 mode=indexing
          tunnel: w241 -> [w293] mode=indexing
          tunnel: [w291] -> w202 mode=indexing
          tunnel: [w290] -> w195 mode=indexing
          n94 = call "getHPData.vi"("HPILC in"=w298) -> ("HPData"=w297:T23)  [unwired: 9 in, 1 out]
          n95 = Unbundle By Name(w297) -> ("Telemetry"=w294:T5, "Telemetry.SSIEncoderValue"=w292:i32, "Telemetry.LoadCellForce"=w290:sgl)
          n96 = Subtract(x=w293, y=w292) -> (x-y=w291:i32)
          n97 = Build Array (concatenate)(w296, w291, w290) -> (w295:dbl[])
        }
        "Actuator Telemetry" <- w244
        n98 = Greater?(x=w162, y=w230) -> (0:w231:bool)
        n99 = Equal?(x=w162, y=w230) -> (x = y?=w240:bool)
        n100 = Quotient & Remainder(x=w162, y=w230) -> (x-y*floor(x/y)=w247:i32)  [unwired: 1 out]
        n101 = case shown="True" w231 {
          tunnel: w229 -> [w272 w281]
          tunnel: [w272 w280] -> w228
          tunnel: w227 -> [_ w273]
          frame False {
          }
          frame True {
            n102 = Unbundle By Name(w281) -> ("MaxLoopTime"=w275:dbl, "MinLoopTime"=w274:dbl)
            n103 = Greater?(x=w273, y=w275) -> (0:w278:bool)
            n104 = Less?(x=w273, y=w274) -> (x < y?=w279:bool)
            n105 = Select(t=w273, s=w278, f=w275) -> (s? t:f=w277:dbl)
            n106 = Select(t=w273, s=w279, f=w274) -> (s? t:f=w276:dbl)
            n107 = Bundle By Name(cluster=w281, "MaxLoopTime"=w277, "MinLoopTime"=w276) -> (w280:T4)
          }
        }
        "output cluster" <- w228
        n108 = Equal To 0?(x=w247) -> (x = 0?=w246:bool)
        n109 = flat-sequence {
          frame #0 {
          }
        }
        n110 = Bundle("Angle"=w170) -> (→"Inclination":cluster{"Angle":sgl})  [unwired: 1 in]
        n111 = case shown="True" w246 {
          tunnel: w207 -> [w286 w288]
          tunnel: [w286 w287] -> w245
          frame False {
          }
          frame True {
            n112 = Multiply(x=w288, y=-1) -> (x*y=w287:i32)
          }
        }
        n113 = Index Array(array=w223, index #1=0 ("index"), index #2=1 ("index"), index #3=2 ("index"), index #4=3 ("index")) -> (element #1=w180:sgl, element #2=w179:sgl, element #3=w178:sgl, element #4=w177:sgl)
        n114 = Index Array(array=w216, index #1=0 ("index"), index #2=1 ("index"), index #3=2 ("index"), index #4=3 ("index"), index #5=4 ("index"), index #6=5 ("index")) -> (element #1=w176:sgl, element #2=w175:sgl, element #3=w174:sgl, element #4=w173:sgl, element #5=w172:sgl, element #6=w171:sgl)
        n115 = case shown="False" w240 {
          tunnel: w243 -> [_ w285]
          tunnel: [w284 w285] -> w242
          tunnel: w241 -> [w284 _]
          frame False {
          }
          frame True {
          }
        }
        n116 = Index Array(array=w202, index #1=0 ("index"), index #2=1 ("index"), index #3=2 ("index"), index #4=3 ("index")) -> (element #1=w196:i32, element #2=w188:i32, element #3=w185:i32, element #4=w182:i32)
        n117 = Index Array(array=w195, index #1=0 ("index"), index #2=1 ("index"), index #3=2 ("index"), index #4=3 ("index")) -> (element #1=w190:sgl, element #2=w187:sgl, element #3=w184:sgl, element #4=w181:sgl)
        n118 = Array To Cluster(array=w234) -> (cluster=→"Encoder":T6)
        n119 = Bundle("Displacement1"=w176, "Displacement1"=w175, "Displacement1"=w174, "Displacement1"=w173, "Displacement1"=w172, "Displacement1"=w171) -> (→"Displacement":T2)  [unwired: 1 in]
        n120 = Bundle("Temperature1"=w180, "Temperature1"=w179, "Temperature1"=w178, "Temperature1"=w177) -> (→"Temperature":T3)  [unwired: 1 in]
        n121 = Format Into String(format string="%d,%d,%d,%f,%d,%d,%f,%d,%d,%f,%d,%d,%f,%f,%f,%f,%f,%f,%f,%f,%f,%f,%f,%f\r\n", w162, w197, w196, w190, w189, w188, w187, w186, w185, w184, w183, w182, w181, w180, w179, w178, w177, w176, w175, w174, w173, w172, w171, w170) -> (resulting string=w169:string)  [unwired: 2 in, 1 out]
        n122 = node-c288() -> ()  [unwired: 1 in, 1 out]
        n123 = Write to Text File(file (use dialog)=w168, text=w169) -> (refnum out=w167:refnum<file>)  [unwired: 2 in, 2 out]
      }
      n124 = node-c288(i64 500 ("Period")) -> (w125:T13)
      n125 = timed-loop {
        timing: w125 -> [_]
        timing-out: [_] -> w124
        shift-right: [w153] -> _
        shift-left: w122 -> [w154]
        stop <- w155 stop-if-true
        n126 = node-c288() -> ()  [unwired: 1 in, 1 out]
        n127 = call "readMonitorAccelerometer.vi"("MonitorAccelerometer in"=w154) -> ("MonitorAccelerometerData"=w148:T44, "MonitorAccelerometer out"=w153:refnum<class "MonitorAccelerometer.lvclass">)  [unwired: 8 in, 1 out]
        n128 = Unbundle By Name(w148) -> ("Timestamp"=w152:dbl[], "Channel0"=w151:sgl[], "Channel1"=w150:sgl[], "Channel2"=w149:sgl[])
        n129 = Bundle("Timestamp"=w152, "Channel0"=w151) -> (w147:cluster{"Timestamp":dbl[], "Channel0":sgl[]})  [unwired: 1 in]
        n130 = Bundle("Timestamp"=w152, "Channel1"=w150) -> (w146:cluster{"Timestamp":dbl[], "Channel1":sgl[]})  [unwired: 1 in]
        n131 = Bundle("Timestamp"=w152, "Channel2"=w149) -> (w145:cluster{"Timestamp":dbl[], "Channel2":sgl[]})  [unwired: 1 in]
        n132 = Build Array(w147, w146, w145) -> (→"XY Graph":cluster{"Timestamp":dbl[], "Channel2":sgl[]}[])
        n133 = local read "Stop"() -> (w155:bool)
        n134 = node-c288() -> ()  [unwired: 1 in, 1 out]
      }
      n135 = node-c288(w124) -> ()  [unwired: 1 out]
      n136 = node-c288(w127) -> ()  [unwired: 1 out]
    }
    frame #3 {
      n137 = Close File(refnum=w322) -> ()  [unwired: 1 in, 2 out]
      n138 = local write "Stop"(FALSE ("Stop")) -> ()
      n139 = xnode "Invoke Method"("FPGA VI Reference In"=w324) -> ("FPGA VI Reference Out"=w325:refnum<k20>)  [unwired: 1 in, 1 out]
      n140 = xnode "Close FPGA VI Reference"("FPGA VI Reference In"=w325) -> ()  [unwired: 1 in, 1 out]
    }
  }
